vi "Processing_Connected_Tracks-11.vi"(0 "[IN] Unsorted \nProblem Tracks":dbl[][](array[numeric]), 1 "[IN] Tracking progress":refnum<vi>, 2 "[IN] Number of SubVI":i32, 3 "[IN] Max angle":dbl, 5 "[IN] Dot matrix \nfor moving points\n(splitted tracks)":i16[][](array[numeric]), 7 "[IN] Potentially\nMoving (X,Y)":dbl[][](array[numeric]), 9 "[IN] Dot matrix with \nstatuses for potentially \nmoving dots":i16[][](array[numeric]), 11 "error IN":errorcluster, 12 "[IN] Primary \n(X,Y) Detected":dbl[][](array[numeric]), 14 "[IN] Areas particles\nPrimary Detected":dbl[][](array[numeric])) -> (4 "[OUT] Before Processing Tracks":T1(array[cluster]), 8 "[OUT] Processed Tracks":T1(array[cluster]), 15 "error OUT":errorcluster)   [LabVIEW 2017]
doc: "Top-level subVI for solving correspondance problems in tracks (in fact, \"tracking\" itself: preserve only 1 track for moving particle)"
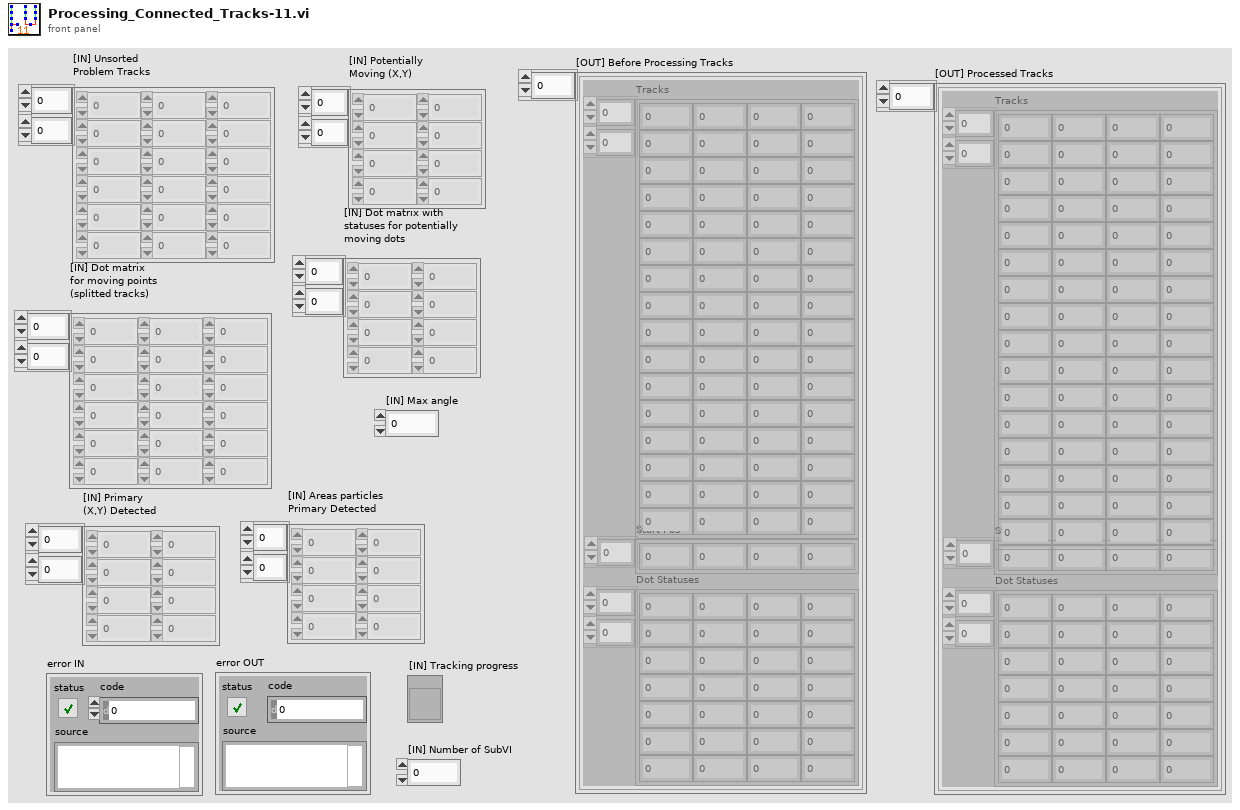
[diagram p1: front panel]
types:
  T1 = cluster{"Tracks":dbl[][], "Start Pos":i32[], "Dot Statuses":i16[][]}[]
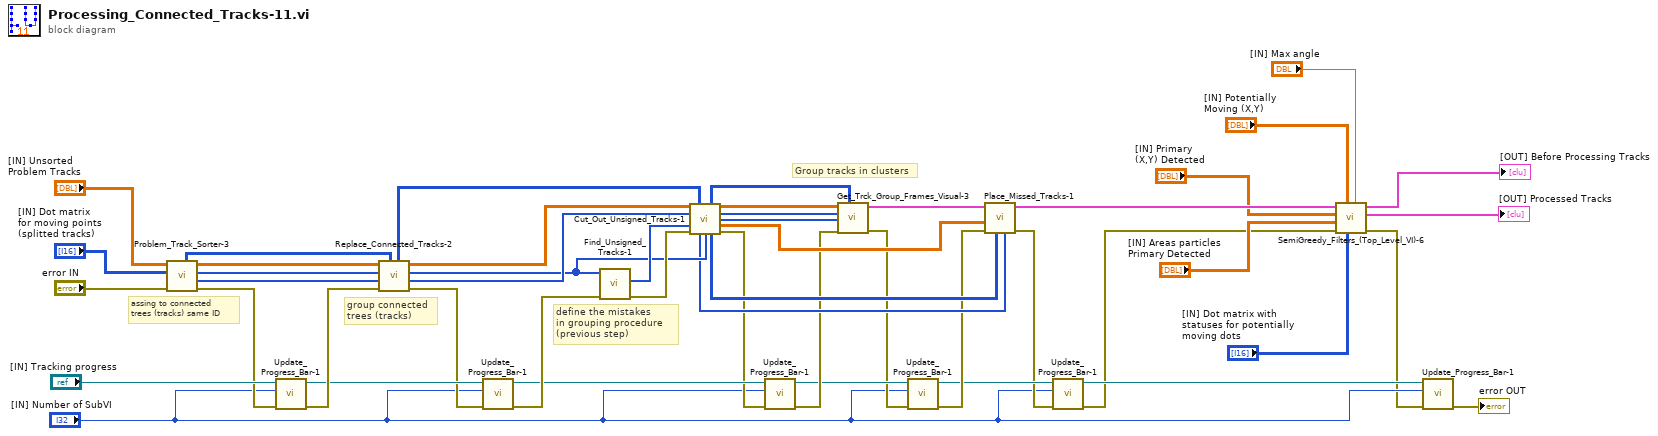
[diagram p0: block diagram]
diagram:
  # "Group tracks in clusters"
  # "define the mistakes\nin grouping procedure \n(previous step)"
  # "group connected\ntrees (tracks)"
  # "assing to connected\ntrees (tracks) same ID"
  n1 = call "Problem_Track_Sorter-3.vi"("[IN] Unsorted Tracks"="[IN] Unsorted \nProblem Tracks", "[IN] Dot matrix"="[IN] Dot matrix \nfor moving points\n(splitted tracks)", "error IN"="error IN") -> ("Filtered Dot Stat Matrix"=w45:i16[][], "Sorted Tracks OUT"=w44:dbl[][], "Track ID OUT"=w43:u16[], "Start Pos OUT"=w42:i32[], "error OUT"=w26:errorcluster)  [unwired: 1 in]
  n2 = call "Update_Progress_Bar-1.vi"("error IN"=w26, "[IN] Number of SubVI"="[IN] Number of SubVI", "[IN] Tracking progress"="[IN] Tracking progress") -> ("error OUT"=w25:errorcluster, "[OUT] Tracking progress"=w24:refnum<vi>)  [unwired: 3 in]
  n3 = call "Replace_Connected_Tracks-2.vi"("Dot Stat Matrix IN"=w45, "error IN"=w25, "Start Pos IN"=w42, "Track ID IN"=w43, "Tracks(PR) IN"=w44) -> ("error OUT"=w23:errorcluster, "Start Pos OUT"=w40:i32[], "Track ID OUT"=w36:u16[], "Tracks(PR) OUT"=w41:dbl[][], "Dot Status OUT"=w37:i16[][])
  n4 = call "Update_Progress_Bar-1.vi"("error IN"=w23, "[IN] Number of SubVI"="[IN] Number of SubVI", "[IN] Tracking progress"=w24) -> ("error OUT"=w22:errorcluster, "[OUT] Tracking progress"=w21:refnum<vi>)  [unwired: 3 in]
  n5 = call "Find_Unsigned_Tracks-1.vi"("error IN"=w22, "Track ID IN"=w36) -> ("error OUT"=w38:errorcluster, "Position Mis ID"=w39:i32[])  [unwired: 3 in, 1 out]
  n6 = call "Cut_Out_Unsigned_Tracks-1.vi"("[IN] Tracks"=w41, "[IN] Dot Status"=w37, "[IN] Start Pos"=w40, "[IN] Position \nof Mistakes"=w39, "error IN"=w38, "[IN] Track ID"=w36) -> ("[OUT] Dot Status"=w32:i16[][], "[OUT] Tracks"=w35:dbl[][], "[OUT] Track ID"=w34:u16[], "[OUT] Start Pos"=w33:i32[], "[OUT] Missed tracks"=w28:dbl[][], "[OUT] Missed Start Pos"=w29:i32[], "[OUT] Missed Dot Status"=w30:i16[][], "error OUT"=w20:errorcluster)  [unwired: 2 in]
  n7 = call "Update_Progress_Bar-1.vi"("error IN"=w20, "[IN] Number of SubVI"="[IN] Number of SubVI", "[IN] Tracking progress"=w21) -> ("error OUT"=w19:errorcluster, "[OUT] Tracking progress"=w18:refnum<vi>)  [unwired: 3 in]
  n8 = call "Get_Trck_Group_Frames_Visual-3.vi"("Dot Status IN"=w32, "error IN"=w19, "Start Pos IN"=w33, "Track ID IN"=w34, "Tracks IN"=w35) -> ("error OUT"=w17:errorcluster, "[OUT] Grou\nped Tracks"=w31:T1)  [unwired: 3 in]
  n9 = call "Update_Progress_Bar-1.vi"("error IN"=w17, "[IN] Number of SubVI"="[IN] Number of SubVI", "[IN] Tracking progress"=w18) -> ("error OUT"=w16:errorcluster, "[OUT] Tracking progress"=w15:refnum<vi>)  [unwired: 3 in]
  n10 = call "Place_Missed_Tracks-1.vi"("[IN] Missed Start Pos"=w29, "[IN] Missed Dot Status"=w30, "error IN"=w16, "[IN] Missed tracks"=w28, "[IN] Before Pro\ncessing Tracks"=w31) -> ("error OUT"=w14:errorcluster, "[OUT] Processed Tracks"=w8:T1)  [unwired: 5 in]
  n11 = call "Update_Progress_Bar-1.vi"("error IN"=w14, "[IN] Number of SubVI"="[IN] Number of SubVI", "[IN] Tracking progress"=w15) -> ("error OUT"=w5:errorcluster, "[OUT] Tracking progress"=w13:refnum<vi>)  [unwired: 3 in]
  n12 = call "SemiGreedy_Filters_(Top_Level_VI)-6.vi"("[IN] Max angle"="[IN] Max angle", "[IN] Dot matrix with statuses \nfor potentially moving dots"="[IN] Dot matrix with \nstatuses for potentially \nmoving dots", "[IN] Possibly\nMoving (X,Y)"="[IN] Potentially\nMoving (X,Y)", "error IN"=w5, "[IN] Areas particles\nPrimary Detected"="[IN] Areas particles\nPrimary Detected", "[IN] Primary \n(X,Y) Detected"="[IN] Primary \n(X,Y) Detected", "[IN] Grouped tracks"=w8) -> ("error OUT"=w3:errorcluster, "[OUT] Processed Tracks"=→"[OUT] Processed Tracks":T1, "[OUT Tracks be\nfore Processing"=→"[OUT] Before Processing Tracks":T1)  [unwired: 2 in]
  n13 = call "Update_Progress_Bar-1.vi"("error IN"=w3, "[IN] Number of SubVI"="[IN] Number of SubVI", "[IN] Tracking progress"=w13) -> ("error OUT"=→"error OUT":errorcluster)  [unwired: 3 in, 1 out]
